vi "ReadCsv.vi"(1 "相对路径":string, 2 "file path (dialog if empty)":path caption="文件路径") -> (0 "all rows":string[][](array[string]) caption="所有行")   [LabVIEW 2018]
uses:
  <vilib>/Utility/file.llb/Read Delimited Spreadsheet (string).vi
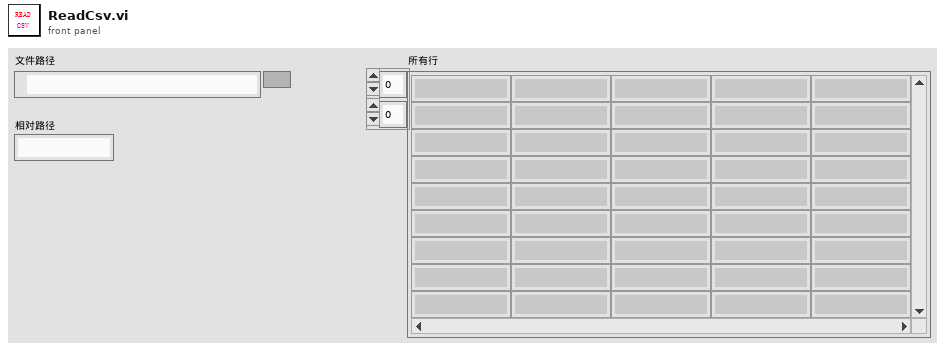
[diagram p1: front panel]
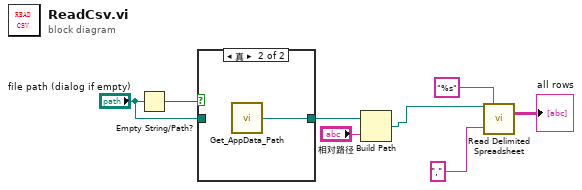
[diagram p0: block diagram]
diagram:
  n1 = Empty String/Path?(string/path="file path (dialog if empty)") -> (empty?=w5:bool)
  n2 = case shown="真" w5 {
    tunnel: [w9 w10] -> w3
    tunnel: "file path (dialog if empty)" -> [w9 _]
    frame False {
    }
    frame True {
      n3 = call "Get_AppData_Path.vi"() -> ("path"=w10:path)  [unwired: 1 in]
    }
  }
  n4 = Build Path(base path=w3, name or relative path="相对路径") -> (appended path=w2:path)
  n5 = call-poly <vilib>:"Read Delimited Spreadsheet.vi"("file path (dialog if empty)"=w2, "format (%s)"="%s", "delimiter (\\t)"="," ("delimiter (\\t)")) -> ("all rows"=→"all rows":string[][])  [unwired: 7 in, 5 out]
